vi "Read Eat time.vi"(8 "error in (no error)":errorcluster, 11 "Star in":refnum<class "Star.lvclass">) -> (0 "error out":errorcluster, 2 "Eat time":timestamp, 3 "Star out":refnum<class "Star.lvclass">)   [LabVIEW 2021, in "Star.lvclass"]
uses:
  Star.lvclass
  Star.lvclass/Star.ctl
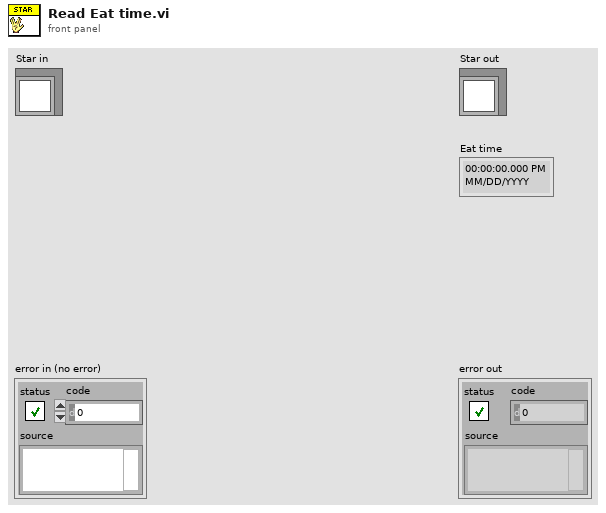
[diagram p1: front panel]
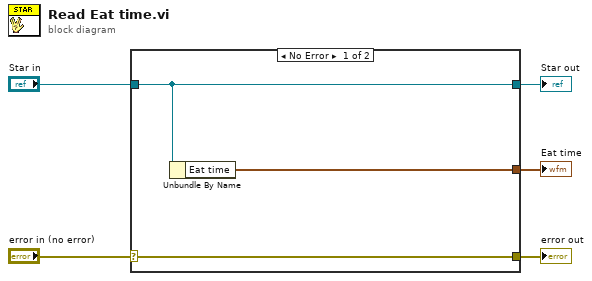
[diagram p0: block diagram]
diagram:
  n1 = case shown="No Error" "error in (no error)" {
    selector: "error in (no error)" -> [w8 w9]
    tunnel: [w8 w9] -> w4
    tunnel: [w7 w10] -> w2
    tunnel: "Star in" -> [w7 w10]
    tunnel: [w6 _] -> w1
    frame No Error {
      n2 = Unbundle By Name(w7) -> ("Eat time"=w6:timestamp)
    }
    frame Error {
    }
  }
  "error out" <- w4
  "Star out" <- w2
  "Eat time" <- w1
